vi "Pcre2MoOfSubstrNumFmOv.vi"(8 "error in":errorcluster, 9 "Number":i32, 11 "pOvector":u64) -> (0 "error out":errorcluster, 1 "OffsetPastMatch":i32, 2 "MatchOffset":i32, 3 "pOvektor":u64 format="%.0x")   [LabVIEW 2021, in "libpcre2-8.lvlib"]
uses:
  libpcre2-8.lvlib
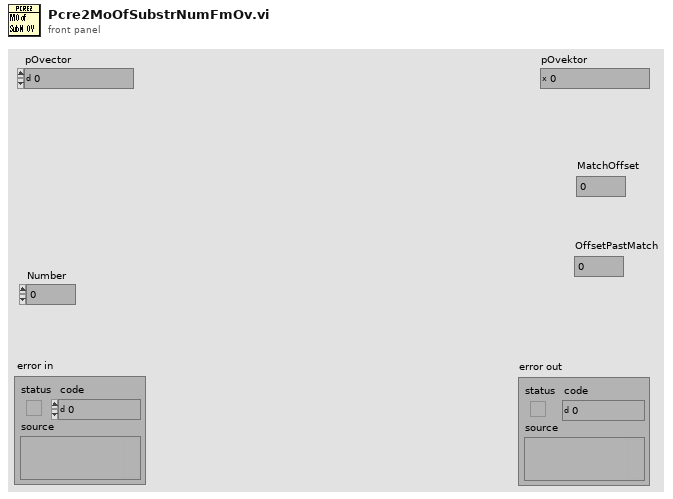
[diagram p1: front panel]
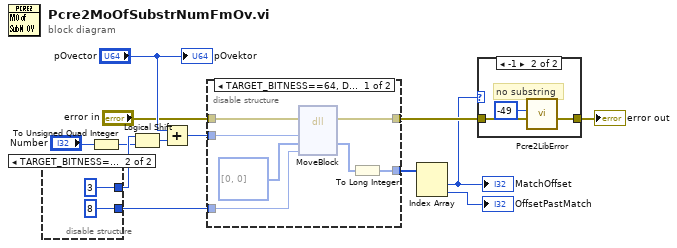
[diagram p0: block diagram]
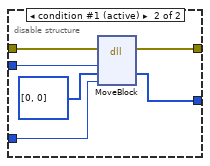
[diagram p3: hidden frame]
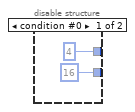
[diagram p4: hidden frame]
diagram:
  n1 = disable-structure shown="TARGET_BITNESS==32" {
    disable-tunnel: [i16 4 ("y") i16 3 ("y")] -> w8
    disable-tunnel: [u64 16 ("y") u64 8 ("y")] -> w9
    frame condition #0 {
    }
    frame condition #1 (active) {
    }
  }
  n2 = To Unsigned Quad Integer(1:"Number") -> (0:w5:u64)
  n3 = Logical Shift(y=w8, x=w5) -> (x << y=w7:u64)
  n4 = Add(x="pOvector", y=w7) -> (x+y=w6:u64)
  n5 = disable-structure shown="TARGET_BITNESS==64, Default" {
    disable-tunnel: w6 -> [w24 w30]
    disable-tunnel: [w23 w29] -> w3
    disable-tunnel: "error in" -> [w22 w28]
    disable-tunnel: [w20 w27] -> w4
    disable-tunnel: w9 -> [w19 w26]
    frame condition #0 {
      n6 = dll-call lib="LabVIEW" fn="MoveBlock"(error in=w22, "pointerSrc"=w24, "pointerDest"=i64[] [0, 0] ("initialized array"), "size"=w19) -> (error out=w23:errorcluster, "pointerDest"=w21:i64[])  [unwired: 5 in, 1 out]
      n7 = To Long Integer(number=w21) -> (32bit integer=w20:i32[])
    }
    frame condition #1 (active) {
      n8 = dll-call lib="LabVIEW" fn="MoveBlock"(error in=w28, "pointerSrc"=w30, "pointerDest"=i32[] [0, 0] ("initialized array"), "size"=w26) -> (error out=w29:errorcluster, "pointerDest"=w27:i32[])  [unwired: 5 in, 1 out]
    }
  }
  n9 = Index Array(array=w4) -> (element #1=w1:i32, element #2=→"OffsetPastMatch":i32)  [unwired: 2 in]
  "MatchOffset" <- w1
  n10 = case shown="-1" w1 {
    tunnel: w3 -> [w31 w33]
    tunnel: [w31 w32] -> w2
    frame Default {
    }
    frame -1 {
      # "no substring"
      n11 = call "Pcre2LibError.vi"("error in"=w33, "ErrorCode"=-49) -> ("error out"=w32:errorcluster)  [unwired: 9 in]
    }
  }
  "error out" <- w2
  "pOvektor" <- "pOvector"
